vi "Black Board Performance test.vi"() -> ()   [LabVIEW 2021]
uses:
  Source/Blackboard/Blackboard.lvclass
  <vilib>/TSA/Abstract Data Classes/Abs_Types/Boolean/Abs_Boolean.lvclass
panel:
  out "Boolean":bool
  out "x/y":dbl format="%#_6p"
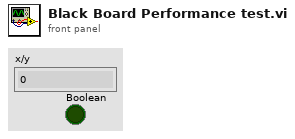
[diagram p1: front panel]
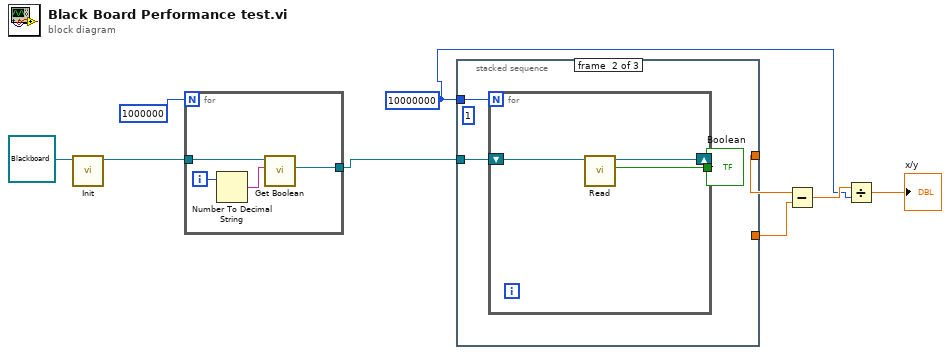
[diagram p0: block diagram]
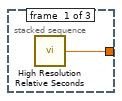
[diagram p2: hidden frame]
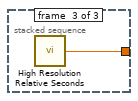
[diagram p3: hidden frame]
diagram:
  w2 = 10000000
  n1 = call-dynamic "Init.vi"("bt_Blackboard in"=refnum<class "Blackboard.lvclass"> refnum) -> ("bt_Blackboard out"=w7:refnum<class "Blackboard.lvclass">)  [unwired: 9 in, 1 out]
  n2 = for {
    N: 1000000 -> [_]
    tunnel: [w12] -> w8
    tunnel: w7 -> [w13]
    i -> [w11]
    n3 = Number To Decimal String(number=w11) -> (decimal integer string=w10:string)  [unwired: 1 in]
    n4 = call "Get Boolean.vi"("Tag"=w10, "Blackboard in"=w13) -> ("Value"=w12:refnum<class "Abs_Boolean.lvclass">)  [unwired: 6 in, 3 out]
  }
  n5 = stacked-sequence {
    tunnel: w8 -> [_ w17 _]
    tunnel: [w14 _ _] -> w4
    tunnel: [_ _ w21] -> w5
    tunnel: w2 -> [_ w16 _]
    frame #0 {
      n6 = call <vilib>:"High Resolution Relative Seconds.vi"() -> ("relative seconds"=w14:dbl)
    }
    frame #1 {
      (unwired) 1
      n7 = for {
        N: w16 -> [_]
        tunnel: [w19] -> w15
        shift-right: [w18] -> _
        shift-left: w17 -> [w20]
        n8 = call-dynamic "Read.vi"("Boolean in"=w20) -> ("Boolean"=w19:bool, "Boolean out"=w18:refnum<class "Abs_Boolean.lvclass">)  [unwired: 8 in, 1 out]
      }
      "Boolean" <- w15
    }
    frame #2 {
      n9 = call <vilib>:"High Resolution Relative Seconds.vi"() -> ("relative seconds"=w21:dbl)
    }
  }
  n10 = Subtract(x=w5, y=w4) -> (x-y=w3:dbl)
  n11 = Divide(x=w3, y=w2) -> (x/y=→"x/y":dbl)
